vi "Update Channel and Objective UI .vi"(8 "error in (no error)":errorcluster, 10 "OME_MD_GUI control references":T1, 11 "DOM document IN":refnum<k20>) -> (0 "error out":errorcluster, 3 "node out":refnum<k20>)   [LabVIEW 2012]
doc: "SciScan 1.2 160622"
uses:
  Custom Controls and Typedefs/Experiment and Experimenter.ctl
  Custom Controls and Typedefs/Objective Parameters Cluster.ctl
  Custom Controls and Typedefs/Channel Parameters Cluster.ctl
  <vilib>/regexp/Match Regular Expression.xnode
  <vilib>/xml/NI_XML.lvlib
  <resource>/objmgr/DOMUserDefRef.rc
panel:
  in  "Objective Parameters":T2[](array[typedef])
  in  "Experiment and Experimenter Details":T3
  # "Experiment"
  # "Experimenter"
  # "Sample"
  # "Experiment"
  # "Experimenter"
  # "Sample"
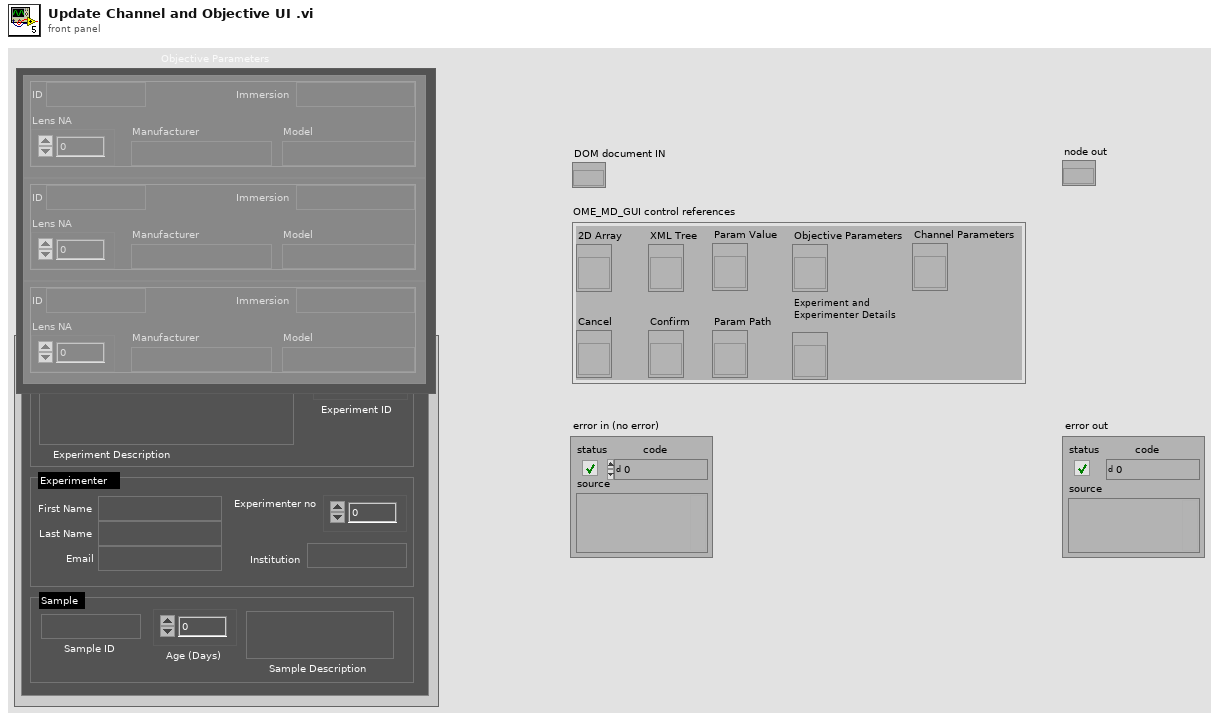
[diagram p1: front panel]
types:
  T1 = cluster{"2D Array":refnum<vi>, "XML Tree":refnum<vi>, "Param Value":refnum<vi>, "Cancel":refnum<vi>, "Confirm":refnum<vi>, "Param Path":refnum<vi>, "Objective Parameters":refnum<vi>, "Experiment and Experimenter Details":refnum<vi>, "Channel Parameters":refnum<vi>}
  T2 = typedef "Objective Parameters Cluster.ctl" = cluster{"ID":string, "Immersion":string, "Lens NA":dbl, "Manufacturer":string, "Model":string}
  T3 = typedef "Experiment and Experimenter.ctl" = cluster{"Experimenter no":u32, "First Name":string, "Experiment ID":string, "urn:lsid: ":string, "Experiment Description":string, "Last Name":string, "Email":string, "Institution":string, "Sample ID":string, "Age (Days)":u32, "Sample Description":string}
  T4 = typedef "Channel Parameters Cluster.ctl" = cluster{"Name (Alias)":string, "ID":string, "Fluor":string, "Colour (RGBA encoded)":i32, "Emission Wavelength":dbl, "Excitation Wavelength":dbl}
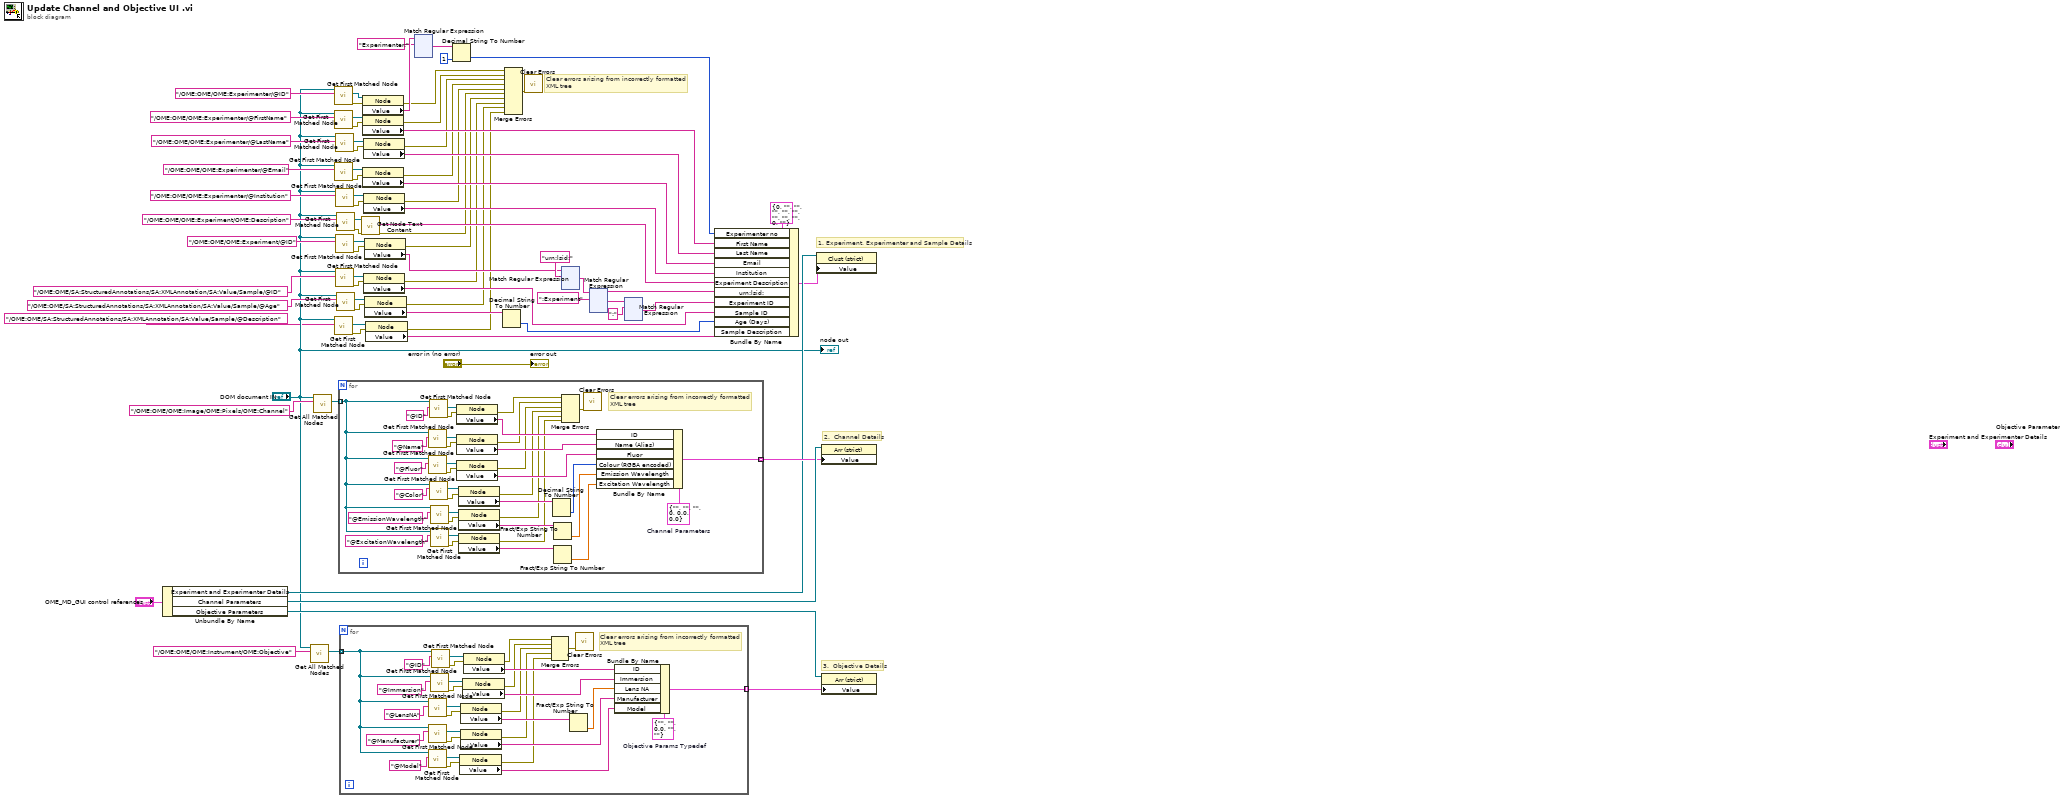
[diagram p0: block diagram]
diagram:
  # "Clear errors arising from incorrectly formatted\nXML tree"
  # "3.  Objective Details"
  # "2.  Channel Details"
  # "1. Experiment, Experimenter and Sample Details"
  n1 = Unbundle By Name("OME_MD_GUI control references") -> ("Experiment and Experimenter Details"=w36:refnum<vi>, "Channel Parameters"=w74:refnum<vi>, "Objective Parameters"=w69:refnum<vi>)
  n2 = call <vilib>:"Get All Matched Nodes.vi"("XPath expression"="/OME:OME/OME:Instrument/OME:Objective", "node in"="DOM document IN") -> ("node result array"=w70:refnum<k20>[])  [unwired: 7 in, 2 out]
  n3 = call <vilib>:"Get All Matched Nodes.vi"("XPath expression"="/OME:OME/OME:Image/OME:Pixels/OME:Channel", "node in"="DOM document IN") -> ("node result array"=w76:refnum<k20>[])  [unwired: 7 in, 2 out]
  n4 = call <vilib>:"Get First Matched Node.vi"("XPath expression"="/OME:OME/SA:StructuredAnnotations/SA:XMLAnnotation/SA:Value/Sample/@Description" ("search string/char (-)"), "node in"="DOM document IN") -> ("error out"=w15:errorcluster, "node result"=w3:refnum<k20>)  [unwired: 7 in, 1 out]
  n5 = call <vilib>:"Get First Matched Node.vi"("XPath expression"="/OME:OME/OME:Experimenter/@ID", "node in"="DOM document IN") -> ("error out"=w32:errorcluster, "node result"=w59:refnum<k20>)  [unwired: 7 in, 1 out]
  n6 = call <vilib>:"Get First Matched Node.vi"("XPath expression"="/OME:OME/OME:Experimenter/@FirstName", "node in"="DOM document IN") -> ("error out"=w31:errorcluster, "node result"=w51:refnum<k20>)  [unwired: 7 in, 1 out]
  n7 = call <vilib>:"Get First Matched Node.vi"("XPath expression"="/OME:OME/OME:Experimenter/@Email", "node in"="DOM document IN") -> ("error out"=w29:errorcluster, "node result"=w47:refnum<k20>)  [unwired: 7 in, 1 out]
  n8 = call <vilib>:"Get First Matched Node.vi"("XPath expression"="/OME:OME/OME:Experimenter/@LastName", "node in"="DOM document IN") -> ("error out"=w30:errorcluster, "node result"=w50:refnum<k20>)  [unwired: 7 in, 1 out]
  n9 = call <vilib>:"Get First Matched Node.vi"("XPath expression"="/OME:OME/SA:StructuredAnnotations/SA:XMLAnnotation/SA:Value/Sample/@ID" ("search string/char (-)"), "node in"="DOM document IN") -> ("error out"=w17:errorcluster, "node result"=w5:refnum<k20>)  [unwired: 7 in, 1 out]
  n10 = call <vilib>:"Get First Matched Node.vi"("XPath expression"="/OME:OME/OME:Experimenter/@Institution", "node in"="DOM document IN") -> ("error out"=w28:errorcluster, "node result"=w46:refnum<k20>)  [unwired: 7 in, 1 out]
  n11 = call <vilib>:"Get First Matched Node.vi"("XPath expression"="/OME:OME/OME:Experiment/@ID", "node in"="DOM document IN") -> ("error out"=w26:errorcluster, "node result"=w66:refnum<k20>)  [unwired: 7 in, 1 out]
  n12 = call <vilib>:"Get First Matched Node.vi"("XPath expression"="/OME:OME/OME:Experiment/OME:Description", "node in"="DOM document IN") -> ("error out"=w27:errorcluster, "node result"=w33:refnum<k20>)  [unwired: 7 in, 1 out]
  n13 = call <vilib>:"Get First Matched Node.vi"("XPath expression"="/OME:OME/SA:StructuredAnnotations/SA:XMLAnnotation/SA:Value/Sample/@Age" ("search string/char (-)"), "node in"="DOM document IN") -> ("error out"=w16:errorcluster, "node result"=w4:refnum<k20>)  [unwired: 7 in, 1 out]
  n14 = for {
    tunnel: w76 -> [w91] mode=indexing
    tunnel: [w92] -> w73 mode=indexing
    w96 = T4 {"Name (Alias)"="", "ID"="", "Fluor"="", "Colour (RGBA encoded)"=0, "Emission Wavelength"=0.0, "Excitation Wavelength"=0.0}  # Channel Parameters
    # "Clear errors arising from incorrectly formatted\nXML tree"
    n15 = call <vilib>:"Get First Matched Node.vi"("XPath expression"="@Name", "node in"=w91) -> ("error out"=w89:errorcluster, "node result"=w110:refnum<k20>)  [unwired: 7 in, 1 out]
    n16 = call <vilib>:"Get First Matched Node.vi"("XPath expression"="@Fluor", "node in"=w91) -> ("error out"=w88:errorcluster, "node result"=w108:refnum<k20>)  [unwired: 7 in, 1 out]
    n17 = call <vilib>:"Get First Matched Node.vi"("XPath expression"="@ID", "node in"=w91) -> ("error out"=w90:errorcluster, "node result"=w113:refnum<k20>)  [unwired: 7 in, 1 out]
    n18 = call <vilib>:"Get First Matched Node.vi"("XPath expression"="@Color", "node in"=w91) -> ("error out"=w87:errorcluster, "node result"=w104:refnum<k20>)  [unwired: 7 in, 1 out]
    n19 = call <vilib>:"Get First Matched Node.vi"("XPath expression"="@EmissionWavelength", "node in"=w91) -> ("error out"=w86:errorcluster, "node result"=w102:refnum<k20>)  [unwired: 7 in, 1 out]
    n20 = call <vilib>:"Get First Matched Node.vi"("XPath expression"="@ExcitationWavelength", "node in"=w91) -> ("error out"=w85:errorcluster, "node result"=w99:refnum<k20>)  [unwired: 7 in, 1 out]
    n21 = property class="Node"(reference=w113, error in=w90) -> (error out=w84:errorcluster, "Value"=w112:string)  [unwired: 1 out]
    n22 = property class="Node"(reference=w110, error in=w89) -> (error out=w83:errorcluster, "Value"=w109:string)  [unwired: 1 out]
    n23 = property class="Node"(reference=w108, error in=w88) -> (error out=w82:errorcluster, "Value"=w106:string)  [unwired: 1 out]
    n24 = property class="Node"(reference=w104, error in=w87) -> (error out=w81:errorcluster, "Value"=w103:string)  [unwired: 1 out]
    n25 = property class="Node"(reference=w102, error in=w86) -> (error out=w80:errorcluster, "Value"=w97:string)  [unwired: 1 out]
    n26 = property class="Node"(reference=w99, error in=w85) -> (error out=w79:errorcluster, "Value"=w98:string)  [unwired: 1 out]
    n27 = Decimal String To Number(string=w103) -> (number=w95:i32)  [unwired: 2 in, 1 out]
    n28 = Fract/Exp String To Number(string=w97) -> (number=w94:dbl)  [unwired: 3 in, 1 out]
    n29 = Fract/Exp String To Number(string=w98) -> (number=w93:dbl)  [unwired: 3 in, 1 out]
    n30 = Merge Errors(w84, w83, w82, w81, w80, w79) -> (w78:errorcluster)
    n31 = call <vilib>:"Clear Errors.vi"("error in (no error)"=w78) -> ()  [unwired: 6 in, 1 out]
    n32 = Bundle By Name(cluster=w96, "ID"=w112, "Name (Alias)"=w109, "Fluor"=w106, "Colour (RGBA encoded)"=w95, "Emission Wavelength"=w94, "Excitation Wavelength"=w93) -> (w92:T4)
  }
  n33 = for {
    tunnel: w70 -> [w129] mode=indexing
    tunnel: [w126] -> w68 mode=indexing
    w142 = T2 {"ID"="", "Immersion"="", "Lens NA"=0.0, "Manufacturer"="", "Model"=""}  # Objective Params Typedef
    # "Clear errors arising from incorrectly formatted\nXML tree"
    n34 = call <vilib>:"Get First Matched Node.vi"("XPath expression"="@Model", "node in"=w129) -> ("error out"=w115:errorcluster, "node result"=w130:refnum<k20>)  [unwired: 7 in, 1 out]
    n35 = call <vilib>:"Get First Matched Node.vi"("XPath expression"="@LensNA", "node in"=w129) -> ("error out"=w117:errorcluster, "node result"=w134:refnum<k20>)  [unwired: 7 in, 1 out]
    n36 = call <vilib>:"Get First Matched Node.vi"("XPath expression"="@Manufacturer", "node in"=w129) -> ("error out"=w116:errorcluster, "node result"=w133:refnum<k20>)  [unwired: 7 in, 1 out]
    n37 = call <vilib>:"Get First Matched Node.vi"("XPath expression"="@Immersion", "node in"=w129) -> ("error out"=w118:errorcluster, "node result"=w140:refnum<k20>)  [unwired: 7 in, 1 out]
    n38 = call <vilib>:"Get First Matched Node.vi"("XPath expression"="@ID", "node in"=w129) -> ("error out"=w119:errorcluster, "node result"=w144:refnum<k20>)  [unwired: 7 in, 1 out]
    n39 = property class="Node"(reference=w130, error in=w115) -> (error out=w121:errorcluster, "Value"=w127:string)  [unwired: 1 out]
    n40 = property class="Node"(reference=w134, error in=w117) -> (error out=w123:errorcluster, "Value"=w136:string)  [unwired: 1 out]
    n41 = property class="Node"(reference=w133, error in=w116) -> (error out=w122:errorcluster, "Value"=w128:string)  [unwired: 1 out]
    n42 = property class="Node"(reference=w140, error in=w118) -> (error out=w124:errorcluster, "Value"=w138:string)  [unwired: 1 out]
    n43 = property class="Node"(reference=w144, error in=w119) -> (error out=w125:errorcluster, "Value"=w141:string)  [unwired: 1 out]
    n44 = Merge Errors(w125, w124, w123, w122, w121) -> (w120:errorcluster)
    n45 = Fract/Exp String To Number(string=w136) -> (number=w135:dbl)  [unwired: 3 in, 1 out]
    n46 = call <vilib>:"Clear Errors.vi"("error in (no error)"=w120) -> ()  [unwired: 6 in, 1 out]
    n47 = Bundle By Name(cluster=w142, "ID"=w141, "Immersion"=w138, "Lens NA"=w135, "Manufacturer"=w128, "Model"=w127) -> (w126:T2)
  }
  n48 = call <vilib>:"Get Node Text Content.vi"("error in (no error)"=w27, "node in"=w33) -> ("error out"=w20:errorcluster, "node text"=w34:string)  [unwired: 7 in, 1 out]
  n49 = property class="Node"(reference=w59, error in=w32) -> (error out=w25:errorcluster, "Value"=w57:string)  [unwired: 1 out]
  n50 = property class="Node"(reference=w51, error in=w31) -> (error out=w24:errorcluster, "Value"=w44:string)  [unwired: 1 out]
  n51 = property class="Node"(reference=w47, error in=w29) -> (error out=w22:errorcluster, "Value"=w39:string)  [unwired: 1 out]
  n52 = property class="Node"(reference=w50, error in=w30) -> (error out=w23:errorcluster, "Value"=w40:string)  [unwired: 1 out]
  n53 = property class="Node"(reference=w46, error in=w28) -> (error out=w21:errorcluster, "Value"=w38:string)  [unwired: 1 out]
  n54 = property class="Node"(reference=w5, error in=w17) -> (error out=w6:errorcluster, "Value"=w10:string)  [unwired: 1 out]
  n55 = property class="Node"(reference=w66, error in=w26) -> (error out=w19:errorcluster, "Value"=w64:string)  [unwired: 1 out]
  n56 = property class="Node"(reference=w4, error in=w16) -> (error out=w2:errorcluster, "Value"=w9:string)  [unwired: 1 out]
  n57 = property class="Node"(reference=w3, error in=w15) -> (error out=w1:errorcluster, "Value"=w7:string)  [unwired: 1 out]
  n58 = xnode "Match Regular Expression"("input string"=w57, "regular expression"="Experimenter:" ("search string/char (-)")) -> ("after match"=w55:string)  [unwired: 4 in, 4 out]
  n59 = Decimal String To Number(string=w55, default (0L)=1 ("default (0 I32)")) -> (number=w53:i32)  [unwired: 1 in, 1 out]
  n60 = Decimal String To Number(string=w9) -> (number=w8:i32)  [unwired: 2 in, 1 out]
  n61 = Merge Errors(w25, w24, w23, w22, w21, w20, w19, w6, w2, w1) -> (w18:errorcluster)
  n62 = call <vilib>:"Clear Errors.vi"("error in (no error)"=w18) -> ()  [unwired: 6 in, 1 out]
  n63 = xnode "Match Regular Expression"("input string"=w64, "regular expression"="urn:lsid:" ("search string/char (-)")) -> ("after match"=w63:string)  [unwired: 4 in, 4 out]
  n64 = xnode "Match Regular Expression"("input string"=w63, "regular expression"=":Experiment" ("search string/char (-)")) -> ("before match"=w60:string, "after match"=w42:string)  [unwired: 4 in, 3 out]
  n65 = xnode "Match Regular Expression"("input string"=w42, "regular expression"=":") -> ("after match"=w37:string)  [unwired: 4 in, 4 out]
  n66 = Bundle By Name(cluster=T3 {"Experimenter no"=0, "First Name"="", "Experiment ID"="", "urn:lsid: "="", "Experiment Description"="", "Last Name"="", "Email"="", "Institution"="", "Sample ID"="", "Age (Days)"=0, "Sample Description"=""} ("Experiment and Experimenter Details"), "Experimenter no"=w53, "First Name"=w44, "Last Name"=w40, "Email"=w39, "Institution"=w38, "Experiment Description"=w34, "urn:lsid:"=w60, "Experiment ID"=w37, "Sample ID"=w10, "Age (Days)"=w8, "Sample Description"=w7) -> (w35:T3)
  n67 = property class="Clust (strict)"(reference=w36, "Value"=w35) -> ()  [unwired: 1 in, 2 out]
  n68 = property class="Arr (strict)"(reference=w74, "Value"=w73) -> ()  [unwired: 1 in, 2 out]
  n69 = property class="Arr (strict)"(reference=w69, "Value"=w68) -> ()  [unwired: 1 in, 2 out]
  "node out" <- "DOM document IN"
  "error out" <- "error in (no error)"
